vi "GetDateReferred.vi"(8 "Error In":errorcluster, 11 "reference in":refnum<class "ReferredBy.lvclass">) -> (0 "Error Out":errorcluster, 2 "DateReferred":timestamp, 3 "reference out":refnum<class "ReferredBy.lvclass">)   [LabVIEW 2020, in "ReferredBy.lvclass"]
uses:
  ReferredBy.lvclass
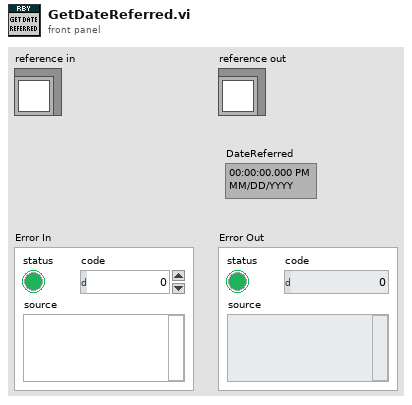
[diagram p1: front panel]
types:
  T1 = typedef "ReferredBy.lvclass/ObjectAttributes.ctl" = cluster{"Customer":refnum<class "Customer.lvclass">, "DateReferred":timestamp}
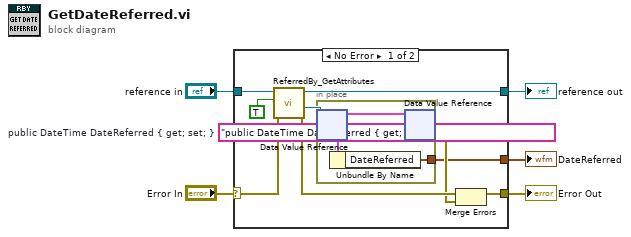
[diagram p0: block diagram]
diagram:
  (unwired) "public DateTime DateReferred { get; set; }"  # public DateTime DateReferred { get; set; }
  n1 = case shown="No Error" "Error In" {
    selector: "Error In" -> [w14 w18]
    tunnel: [w12 w18] -> w4
    tunnel: [w9 w17] -> w2
    tunnel: "reference in" -> [w10 w17]
    tunnel: [w6 _] -> w1
    frame No Error {
      n2 = call "ReferredBy_GetAttributes.vi"("error in (no error)"=w14, "OnlyGetDvrReference(False)"=TRUE, "reference in"=w10) -> ("error out"=w13:errorcluster, "DataRef"=w7:refnum<data-value>, "reference out"=w9:refnum<class "ReferredBy.lvclass">)  [unwired: 5 in, 1 out]
      n3 = in-place {
        in-place-border: [w16] -> w6
        n4 = in-place-dvr #1(w7) -> (w15:T1)  [unwired: 1 out]
        n5 = Unbundle By Name(w15) -> ("DateReferred"=w16:timestamp)
        n6 = in-place-dvr #1(w15) -> (w11:errorcluster)  [unwired: 1 out]
      }
      n7 = Merge Errors(w13, w11) -> (w12:errorcluster)
    }
    frame Error {
    }
  }
  "Error Out" <- w4
  "reference out" <- w2
  "DateReferred" <- w1
